vi "Data.vi"() -> ()   [LabVIEW 2013]
panel:
  in  "Data":dbl[][](array[numeric])
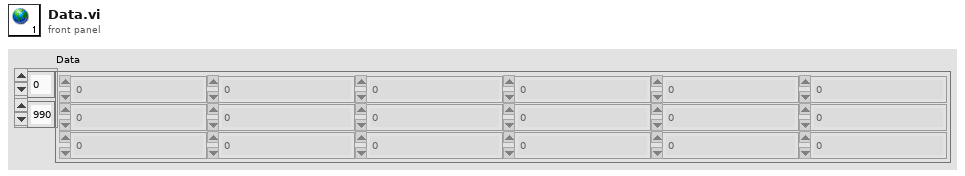
[diagram p1: front panel]
diagram:
